vi "Add to Listbox.vi"() -> ()   [LabVIEW 2019]
uses:
  <vilib>/NI VeriStand/Custom Device API/Custom Device API.lvlib
  <vilib>/NI VeriStand/Custom Device Tools/Custom Device Utility Library/Custom Device Utility Library.lvlib
  FPGA Addon System Explorer.lvlib
  <vilib>/NI VeriStand/Custom Device API/Custom Device Item Ref.ctl
  Listbox Cluster.ctl
panel:
  out "Cluster out":T1 {"Section Ref" format="%.0x"}
  in  "Cluster":T1 {"Section Ref" format="%.0x"}
  out "error out":errorcluster
  in  "error in (no error)":errorcluster
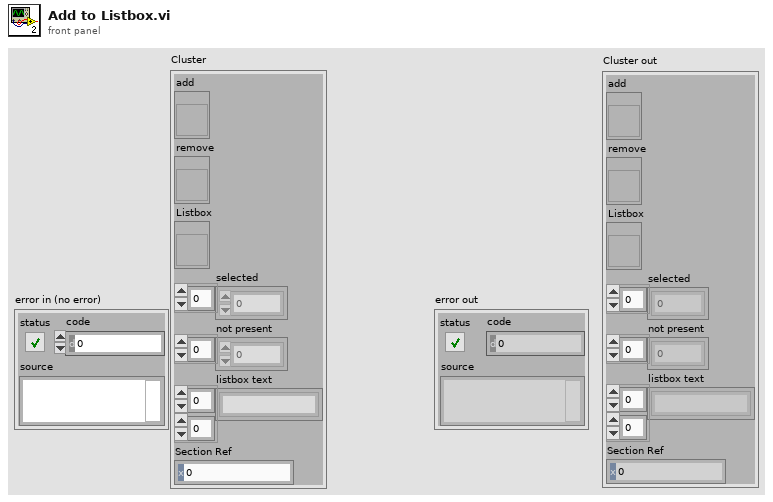
[diagram p1: front panel]
types:
  T1 = typedef "FPGA Addon System Explorer.lvlib/Listbox Cluster.ctl" = cluster{"add":refnum<vi>, "remove":refnum<vi>, "Listbox":refnum<vi>, "selected":i32[], "not present":i32[], "listbox text":string[][], "Section Ref":T2}
  T2 = typedef "Custom Device API.lvlib/Custom Device Item Ref.ctl" = u64
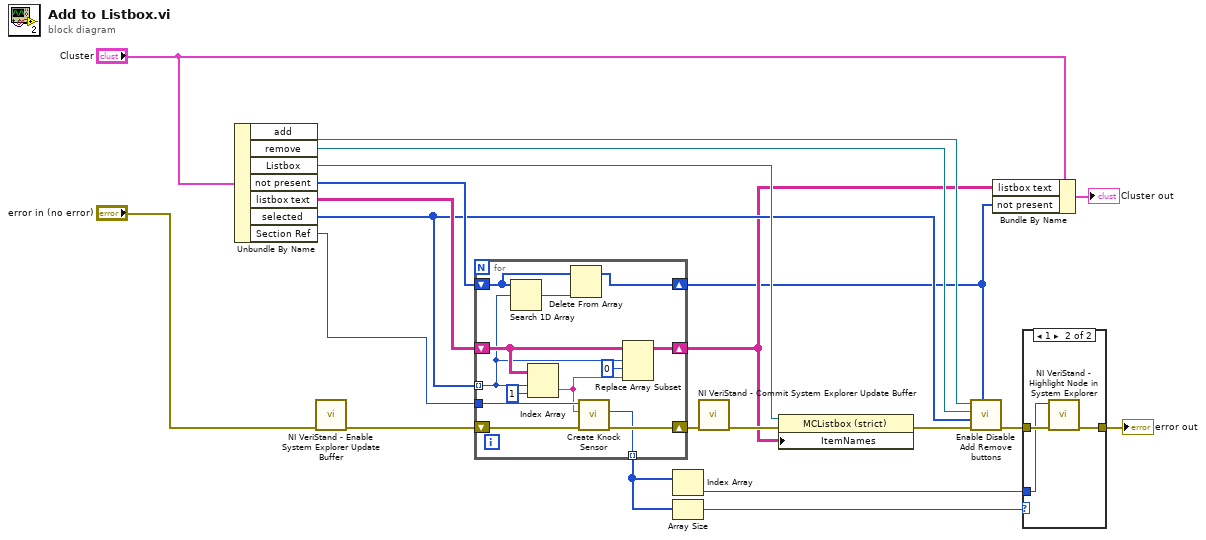
[diagram p0: block diagram]
diagram:
  n1 = Unbundle By Name("Cluster") -> ("add"=w7:refnum<vi>, "remove"=w12:refnum<vi>, "Listbox"=w11:refnum<vi>, "not present"=w8:i32[], "listbox text"=w9:string[][], "selected"=w5:i32[], "Section Ref"=w10:T2)
  n2 = call <vilib>:"NI VeriStand - Enable System Explorer Update Buffer.vi"("error in (no error)"="error in (no error)") -> ("error out"=w14:errorcluster)  [unwired: 10 in]
  n3 = for {
    tunnel: w10 -> [w32]
    shift-right: [w33] -> w21
    shift-left: w14 -> [w34]
    tunnel: w5 -> [w26] mode=indexing
    shift-right: [w29] -> w4
    shift-left: w9 -> [w30]
    shift-right: [w23] -> w3
    shift-left: w8 -> [w25]
    tunnel: [w22] -> w18 mode=indexing
    n4 = Search 1D Array(1D array=w25, element=w26) -> (index of element=w24:i32)  [unwired: 1 in]
    n5 = Index Array(array=w30, index (row)=w26, index (col)=1 ("disabled index (col)")) -> (element=w27:string)
    n6 = Delete From Array(array=w25, index=w24) -> (array with subset deleted=w23:i32[])  [unwired: 1 in, 1 out]
    n7 = call "Create Knock Sensor.vi"("error in (no error)"=w34, "knock sensor name"=w27, "Section Ptr"=w32) -> ("error out"=w33:errorcluster, "Knock sensor ref"=w22:T2)  [unwired: 6 in, 1 out]
    n8 = Replace Array Subset(array=w30, new element=w27, index (row)=w26, index (col)=0 ("disabled index (col)")) -> (w29:string[][])
  }
  n9 = Index Array(array=w18) -> (element=w15:T2)  [unwired: 1 in]
  n10 = Array Size(array=w18) -> (size(s)=w17:i32)
  n11 = call <vilib>:"NI VeriStand - Commit System Explorer Update Buffer.vi"("error in (no error)"=w21) -> ("error out"=w19:errorcluster)  [unwired: 10 in]
  n12 = property on="Property Node" class="MCListbox (strict)"(reference=w11, error in=w19, "ItemNames"=w4) -> (error out=w20:errorcluster)  [unwired: 1 out]
  n13 = call "Enable Disable Add Remove buttons.vi"("not present item indexes"=w3, "error in (no error)"=w20, "selected items"=w5, "remove button"=w12, "add button"=w7) -> ("error out"=w16:errorcluster)  [unwired: 6 in]
  n14 = Bundle By Name(cluster="Cluster", "listbox text"=w4, "not present"=w3) -> (→"Cluster out":T1)
  n15 = case shown="1" w17 {
    tunnel: [w35 w37] -> w1
    tunnel: w16 -> [w35 w38]
    tunnel: w15 -> [_ w36]
    frame Default {
    }
    frame 1 {
      n16 = call <vilib>:"NI VeriStand - Highlight Node in System Explorer.vi"("error in (no error)"=w38, "Item Ref in"=w36) -> ("error out"=w37:errorcluster)  [unwired: 8 in, 1 out]
    }
  }
  "error out" <- w1
